vi "PathPlanner_Path_SamplePath.vi"(9 "Waypoints":T2[](array[typedef]) {"nextControl"."Y" format="%14.3f"; "nextControl"."X" format="%14.3f"; "anchor"."Y" format="%14.3f"; "anchor"."X" format="%14.3f"; "prevControl"."Y" format="%14.3f"; "prevControl"."X" format="%14.3f"}, 11 "WaypointRelativePos":dbl) -> (3 "Sample":T1 {"Y" format="%14.3f"; "X" format="%14.3f"})   [LabVIEW 2019, in "PathPlanner24.lvlib"]
doc: "Get the number of points in this path\n\nInputs: \n - Path - cluster - path definition data structure\n\nOutputs:\n - NumPoints - integer - Number of points in the path"
uses:
  PathPlanner24.lvlib
  TypeDef/PathPlannerWaypoint.ctl
  <vilib>/Rock Robotics/WPI/ThirdParty/JAS_Junk/TrajLib/TypeDef/TRANSLATION2D.ctl
  <vilib>/Rock Robotics/WPI/ThirdParty/JAS_Junk/TrajLib/Trajectory_Library.lvlib
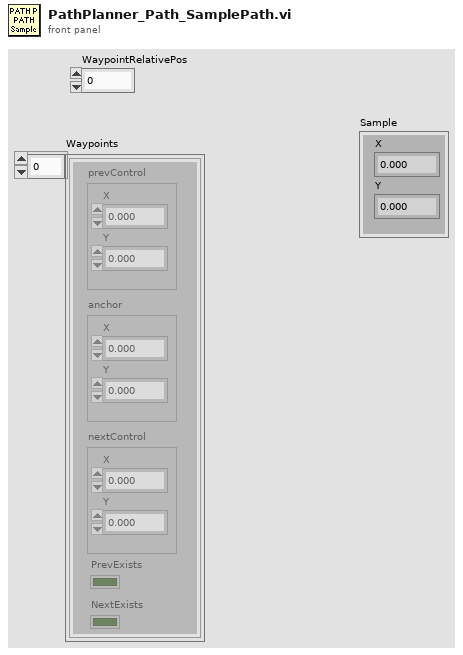
[diagram p1: front panel]
types:
  T1 = typedef "Trajectory_Library.lvlib/TRANSLATION2D.ctl" = cluster{"X":dbl, "Y":dbl}
  T2 = typedef "PathPlanner24.lvlib/PathPlannerWaypoint.ctl" = cluster{"prevControl":T1, "anchor":T1, "nextControl":T1, "PrevExists":bool, "NextExists":bool}
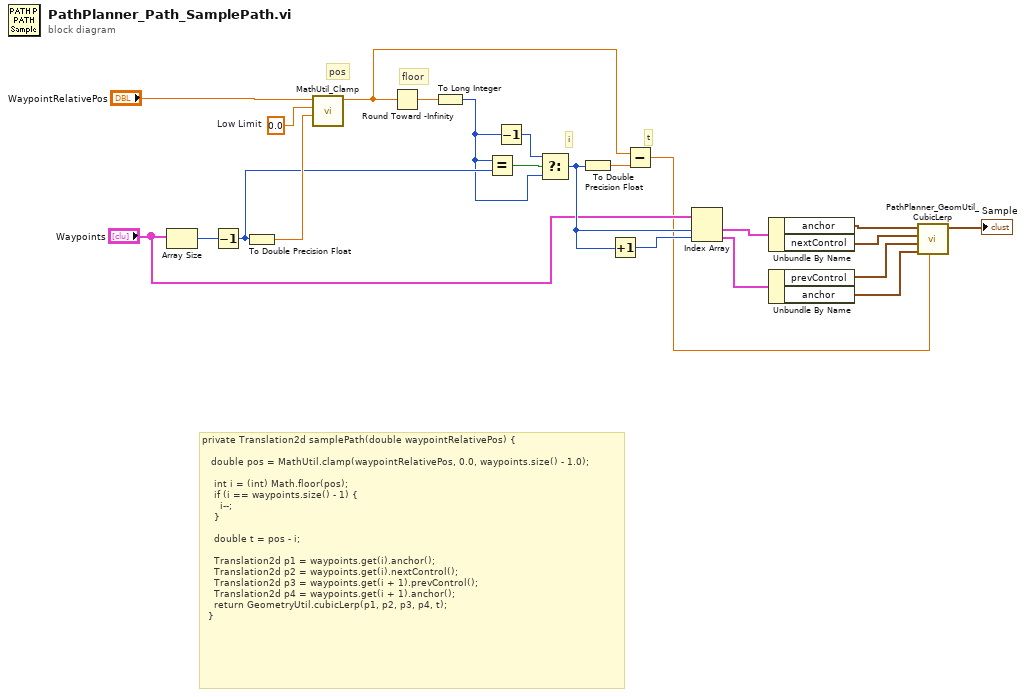
[diagram p0: block diagram]
diagram:
  w22 = 0.0  # Low Limit
  # "i"
  # "t"
  # "floor"
  # "private Translation2d samplePath(double waypointRelativePos) {\n    \n   double pos = MathUtil.clamp(waypointRelativePos, 0.0, waypoints.size() - 1.0);\n\n    int i = (int) Math.floor(pos);\n    if (i == waypoints.size() - 1) {\n      i--;\n    }\n\n    double t = pos - i;\n\n    Translation2d p1 = waypoints.get(i).anchor();\n    Translation2d p2 = waypoints.get(i).nextControl();\n    Translation2d p3 = waypoints.get(i + 1).prevControl();\n    Translation2d p4 = waypoints.get(i + 1).anchor();\n    return GeometryUtil.cubicLerp(p1, p2, p3, p4, t);\n  }"
  # "pos"
  n1 = Array Size(array="Waypoints") -> (size(s)=w20:i32)
  n2 = Decrement(x=w20) -> (x-1=w18:i32)
  n3 = To Double Precision Float(number=w18) -> (double precision float=w19:dbl)
  n4 = call <vilib>:"MathUtil_Clamp.vi"("High Limit"=w19, "Low Limit"=w22, "Value"="WaypointRelativePos") -> ("Result"=w12:dbl)  [unwired: 8 in]
  n5 = Round Toward -Infinity(1:w12) -> (0:w17:dbl)
  n6 = To Long Integer(number=w17) -> (32bit integer=w15:i32)
  n7 = Equal?(x=w15, y=w18) -> (x = y?=w16:bool)
  n8 = Decrement(x=w15) -> (x-1=w14:i32)
  n9 = Select(t=w14, s=w16, f=w15) -> (s? t:f=w11:i32)
  n10 = To Double Precision Float(number=w11) -> (double precision float=w13:dbl)
  n11 = Increment(x=w11) -> (x+1=w10:i32)
  n12 = Subtract(x=w12, y=w13) -> (x-y=w2:dbl)
  n13 = Index Array(array="Waypoints", index #1=w11, index #2=w10) -> (element #1=w8:T2, element #2=w7:T2)
  n14 = Unbundle By Name(w8) -> ("anchor"=w6:T1, "nextControl"=w5:T1)
  n15 = Unbundle By Name(w7) -> ("prevControl"=w4:T1, "anchor"=w3:T1)
  n16 = call "PathPlanner_GeomUtil_CubicLerp.vi"("T"=w2, "D"=w3, "C"=w4, "B"=w5, "A"=w6) -> ("Lerp"=→"Sample":T1)  [unwired: 6 in]
